vi "Read Door Hardware.vi"(11 "Door Controller in":refnum<class "Door Controller.lvclass">) -> (2 "Door Hardware":refnum<class "Message Enqueuer.lvclass">)   [LabVIEW 2020, in "Door Controller.lvlib" / "Door Controller.lvclass"]
uses:
  Door Controller.lvclass
  <vilib>/ActorFramework/Message Enqueuer/Message Enqueuer.lvclass
  Door Controller.lvclass/Door Controller.ctl
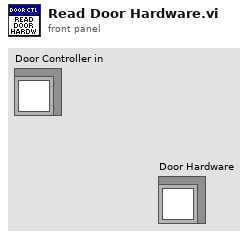
[diagram p1: front panel]
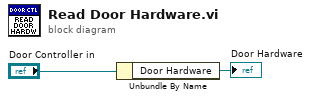
[diagram p0: block diagram]
diagram:
  n1 = Unbundle By Name("Door Controller in") -> ("Door Hardware"=→"Door Hardware":refnum<class "Message Enqueuer.lvclass">)
